vi "Start Server.vi"(8 "error in (no error)":errorcluster, 11 "Server in":refnum<class "Server.lvclass">) -> (0 "error out":errorcluster, 3 "Server out":refnum<class "Server.lvclass">)   [LabVIEW 2013, in "MQTT Server.lvlib" / "Server.lvclass"]
uses:
  Server.lvclass
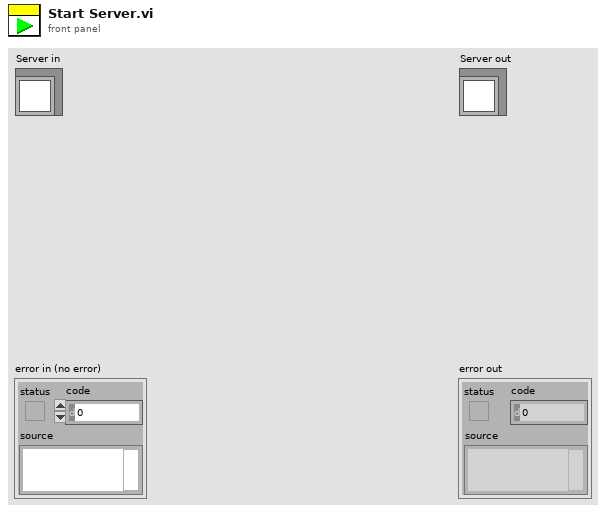
[diagram p1: front panel]
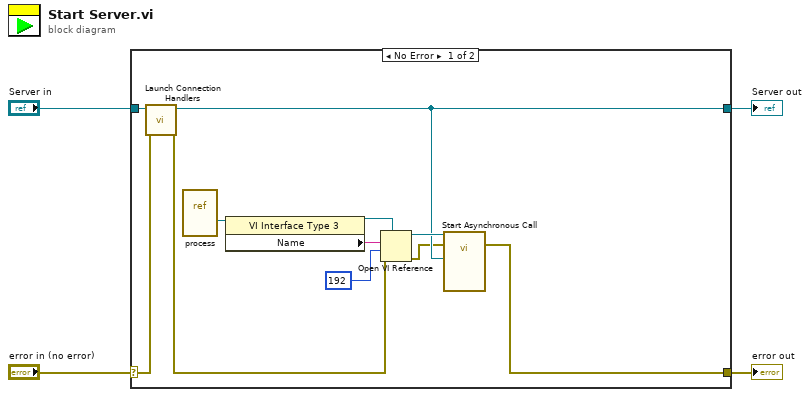
[diagram p0: block diagram]
diagram:
  n1 = case shown="No Error" "error in (no error)" {
    selector: "error in (no error)" -> [w6 w17]
    tunnel: [w7 w17] -> w3
    tunnel: [w10 w16] -> w1
    tunnel: "Server in" -> [w15 w16]
    frame No Error {
      n2 = call "Launch Connection Handlers.vi"("error in (no error)"=w6, "Server in"=w15) -> ("error out"=w5:errorcluster, "Server out"=w10:refnum<class "Server.lvclass">)  [unwired: 8 in]
      n3 = vi-ref "process.vi"() -> (w14:refnum<vi>)
      n4 = property class="VI Interface Type 3"(reference=w14) -> (reference out=w12:refnum<vi>, "Name"=w13:string)  [unwired: 1 in, 1 out]
      n5 = Open VI Reference(type specifier VI Refnum (for type only)=w12, vi path=w13, options=192, error in (no error)=w5) -> (vi reference=w11:refnum<vi>, error out=w9:errorcluster)  [unwired: 2 in]
      n6 = call-by-ref "Start Asynchronous Call"(reference=w11, error in=w9, "Server in"=w10) -> (error out=w7:errorcluster)  [unwired: 9 in, 3 out]
    }
    frame Error {
    }
  }
  "error out" <- w3
  "Server out" <- w1
